vi "Set Cluster Element by Name__ogtk.vi"(8 "error in (no error)":errorcluster, 9 "Element Name (\"\": New Element Data Name)":string, 10 "New Element Value":variant, 11 "Cluster":variant) -> (0 "error out":errorcluster, 1 "found?":bool, 3 "VCluster out":variant)   [LabVIEW 2016]
doc: "Returns a cluster with element replaced with new element value. If <B>Element name</B> unwired, <B>New Element Value</B> data name is used. Data type of the new element is not checked for compatibility with replaced element."
panel:
  # "[OpenG VI Tags] ***Do Not Remove***"
  # "Set Cluster Element by Name.vi\n\nReturns a cluster with element replaced with new element value. If <B>Element na\n\nPlease visit http://www.OpenG.org to learn about the\nOpen Source LabVIEW software movement.\n\nNOTICE -- YOU MUST LEAVE THIS NOTICE IN PLACE.  PER THE TERMS OF THE LICENSE BELOW, YOU MAY SUBLICENSE THIS SOFTWARE \nIN ANY WAY THAT DOES NOT CONFLICT WITH THIS LICENSE.\n\n### BSD License (http://www.opensource.org/licenses/bsd-license.php) Begin ###\n \nCopyright (c) 2002, Jean-Pierre Drolet <drolet_jp@hotmail.com>\nCopyright (c) 2002-2006, Jim Kring <jim@jimkring.com>\n\nAll rights reserved.\n\nRedistribution and use in source and binary forms, with or without modification, are permitted provided that the following conditions are met:\n\n    * Redistributions of source code must retain the above copyright notice, this list of conditions and the following disclaimer.\n    * Redistributions in binary form must reproduce the above copyright notice, this list of conditions and the following disclaimer in the \n       documentation and/or other materials provided with the distribution.\n    * Neither the name of SciWare, James Kring, Inc., nor the names of its contributors may be used to endorse or promote products derived \n       from this software without specific prior written permission.\n\nTHIS SOFTWARE IS PROVIDED BY THE COPYRIGHT HOLDERS AND CONTRIBUTORS \"AS IS\" AND ANY EXPRESS OR IMPLIED WARRANTIES, \nINCLUDING, BUT NOT LIMITED TO, THE IMPLIED WARRANTIES OF MERCHANTABILITY AND FITNESS FOR A PARTICULAR PURPOSE ARE \nDISCLAIMED. IN NO EVENT SHALL THE COPYRIGHT OWNER OR CONTRIBUTORS BE LIABLE FOR ANY DIRECT, INDIRECT, INCIDENTAL,\n SPECIAL, EXEMPLARY, OR CONSEQUENTIAL DAMAGES (INCLUDING, BUT NOT LIMITED TO, PROCUREMENT OF SUBSTITUTE GOODS OR \nSERVICES; LOSS OF USE, DATA, OR PROFITS; OR BUSINESS INTERRUPTION) HOWEVER CAUSED AND ON ANY THEORY OF LIABILITY, \nWHETHER IN CONTRACT, STRICT LIABILITY, OR TORT (INCLUDING NEGLIGENCE OR OTHERWISE) ARISING IN ANY WAY OUT OF THE USE \nOF THIS SOFTWARE, EVEN IF ADVISED OF THE POSSIBILITY OF SUCH DAMAGE.\n\n### BSD License End ###"
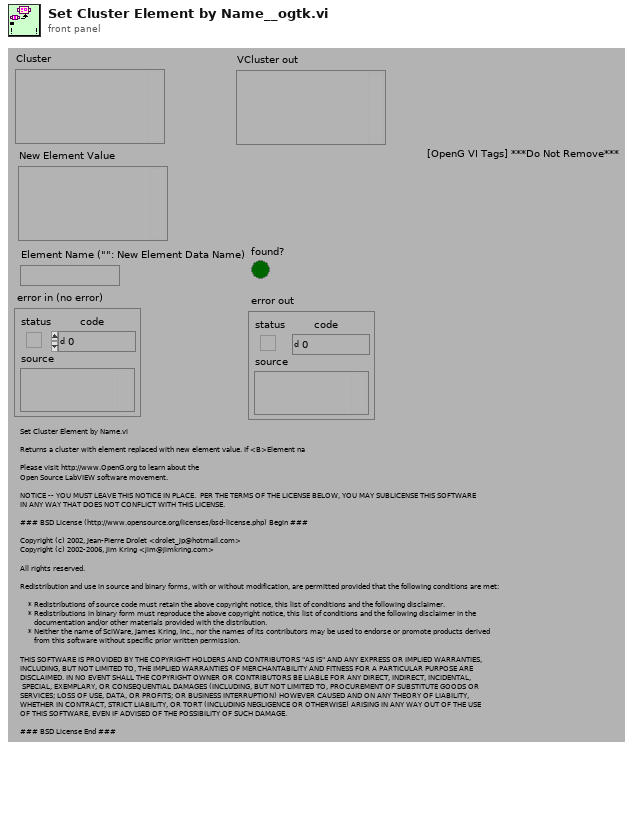
[diagram p1: front panel]
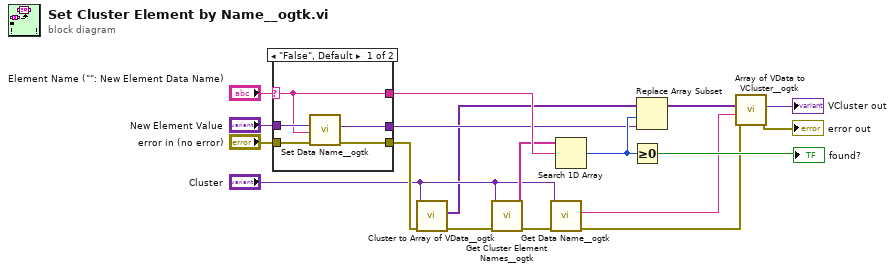
[diagram p0: block diagram]
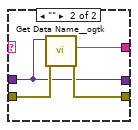
[diagram p2: hidden frame]
diagram:
  n1 = case shown="\"False\", Default" "Element Name (\"\": New Element Data Name)" {
    selector: "Element Name (\"\": New Element Data Name)" -> [w21 _]
    tunnel: "New Element Value" -> [w23 w24]
    tunnel: [w21 w27] -> w12
    tunnel: [w22 w24] -> w3
    tunnel: "error in (no error)" -> [w20 w26]
    tunnel: [w19 w25] -> w13
    frame "False", Default {
      n2 = call "Set Data Name__ogtk.vi"("error in (no error)"=w20, "Data Name"=w21, "Data"=w23) -> ("error out"=w19:errorcluster, "Renamed Data"=w22:variant)  [unwired: 7 in]
    }
    frame "" {
      n3 = call "Get Data Name__ogtk.vi"("error in (no error)"=w26, "Data"=w24) -> ("error out"=w25:errorcluster, "Data Name"=w27:string)  [unwired: 7 in, 1 out]
    }
  }
  n4 = call "Cluster to Array of VData__ogtk.vi"("error in (no error)"=w13, "Cluster"="Cluster") -> ("error out"=w9:errorcluster, "Array of VData"=w2:variant[])  [unwired: 8 in]
  n5 = call "Get Cluster Element Names__ogtk.vi"("error in (no error)"=w9, "Cluster"="Cluster") -> ("error out"=w7:errorcluster, "Element Names"=w8:string[])  [unwired: 8 in]
  n6 = call "Get Data Name__ogtk.vi"("error in (no error)"=w7, "Data"="Cluster") -> ("error out"=w6:errorcluster, "Data Name"=w4:string)  [unwired: 7 in, 1 out]
  n7 = Search 1D Array(1D array=w8, element=w12) -> (index of element=w18:i32)  [unwired: 1 in]
  n8 = Greater Or Equal To 0?(x=w18) -> (x >= 0?=→"found?":bool)
  n9 = Replace Array Subset(array=w2, new element=w3, index=w18) -> (w1:variant[])
  n10 = call "Array of VData to VCluster__ogtk.vi"("error in (no error)"=w6, "Cluster Name"=w4, "Array"=w1) -> ("error out"=→"error out":errorcluster, "VCluster"=→"VCluster out":variant)  [unwired: 7 in]
